vi "FPGA1_EPTDigChannels_ECS.vi"(0 "NI9411-1.2.Filt":u16, 1 "NI9411-1.3.Filt":u16, 2 "NI9411-1.4.Filt":u16, 3 "NI9411-1.5.Filt":u16, 4 "ADCombo-1.VRHallData":T1, 5 "ADCombo-1.VR1.Filt":u16, 6 "ADCombo-1.VR2.Filt":u16, 8 "9411/DI5:0":u8, 9 "ADCombo-1.Hall1.Filt":u16, 10 "NI9411-1.1.Filt":u16, 11 "ADCombo-1.Hall2.Filt":u16, 12 "NI9411-1.Invert":u8, 13 "ADCombo-1.VRHallInvert":u8, 14 "NI9411-1.0.Filt":u16) -> (16 "9411-1.0.PPWData":T2, 17 "ADCombo-1.Hall2.PPWData":T2, 18 "9411-1.1.PPWData":T2, 19 "ADCombo-1.Hall1.PPWData":T2, 20 "9411-1.2.PPWData":T2, 21 "9411-1.3.PPWData":T2, 22 "9411-1.4.PPWData":T2, 23 "9411-1.5.PPWData":T2, 24 "9411-1.DigitalTriggers":bool[](array[boolean]), 25 "ADCombo-1.VR1.PPWData":T2, 26 "ADCombo-1.VR2.PPWData":T2, 27 "ADCombo-1.DigitalTriggers":bool[](array[boolean]))   [LabVIEW 2015, in "ECS-FPGA.lvlib"]
uses:
  ECS-FPGA.lvlib
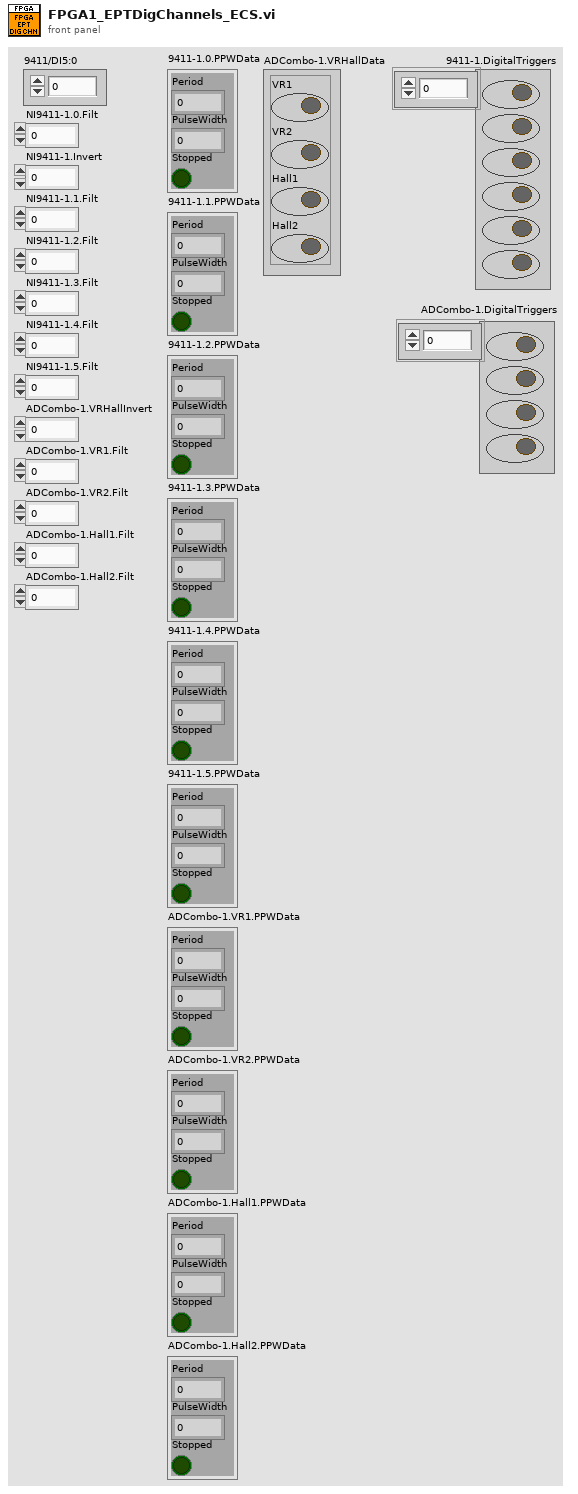
[diagram p1: front panel]
types:
  T1 = cluster{"VR1":bool, "VR2":bool, "Hall1":bool, "Hall2":bool}
  T2 = cluster{"Period":u32, "PulseWidth":u32, "Stopped":bool}
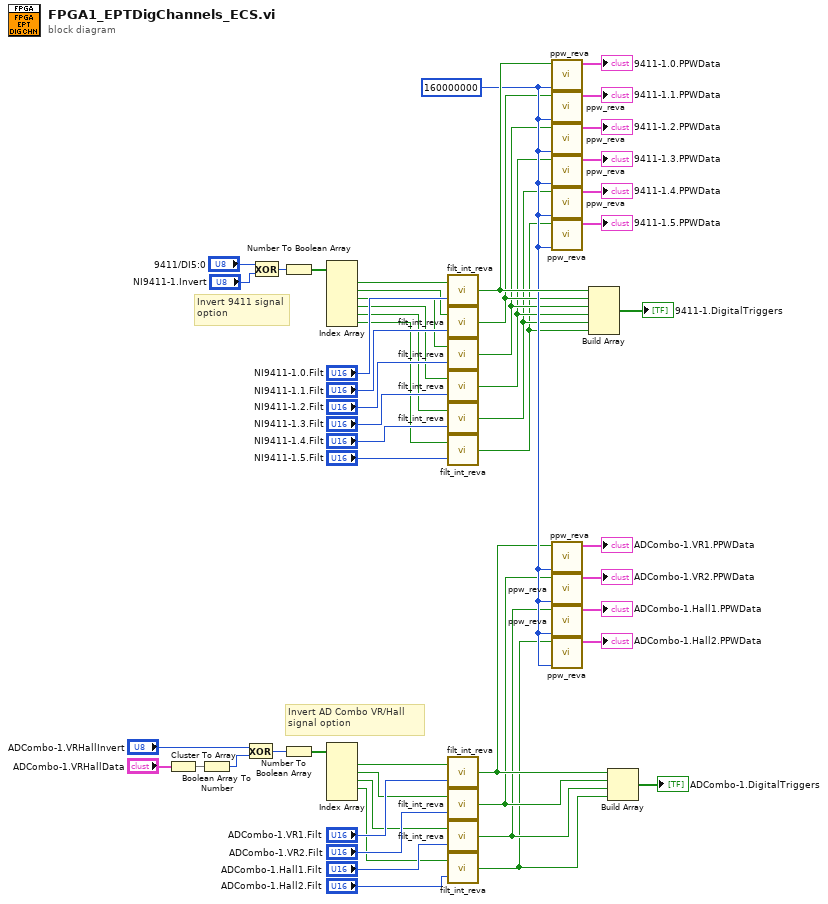
[diagram p0: block diagram]
diagram:
  w48 = u32 160000000 ("StopValue")
  # "Invert AD Combo VR/Hall\nsignal option"
  # "Invert 9411 signal\noption"
  n1 = Cluster To Array(cluster="ADCombo-1.VRHallData") -> (array=w14:bool[])
  n2 = Boolean Array To Number(Boolean array=w14) -> (number=w13:u8)
  n3 = Exclusive Or(1:w13, 2:"ADCombo-1.VRHallInvert") -> (0:w11:u8)
  n4 = Exclusive Or(1:"NI9411-1.Invert", 2:"9411/DI5:0") -> (0:w21:u8)
  n5 = Number To Boolean Array(number=w21) -> (Boolean array=w23:bool[])
  n6 = Number To Boolean Array(number=w11) -> (Boolean array=w9:bool[])
  n7 = Index Array(array=w23) -> (element #1=w24:bool, element #2=w25:bool, element #3=w26:bool, element #4=w27:bool, element #5=w28:bool, element #6=w29:bool)  [unwired: 6 in]
  n8 = Index Array(array=w9) -> (element #1=w10:bool, element #2=w8:bool, element #3=w7:bool, element #4=w6:bool)  [unwired: 5 in, 1 out]
  n9 = call <vilib>:"filt_int_reva.vi"("FiltValue"="NI9411-1.0.Filt", "InpSig"=w24) -> ("OutSig"=w53:bool)
  n10 = call <vilib>:"filt_int_reva.vi"("FiltValue"="NI9411-1.1.Filt", "InpSig"=w25) -> ("OutSig"=w20:bool)
  n11 = call <vilib>:"filt_int_reva.vi"("FiltValue"="NI9411-1.2.Filt", "InpSig"=w26) -> ("OutSig"=w19:bool)
  n12 = call <vilib>:"filt_int_reva.vi"("FiltValue"="NI9411-1.3.Filt", "InpSig"=w27) -> ("OutSig"=w18:bool)
  n13 = call <vilib>:"filt_int_reva.vi"("FiltValue"="NI9411-1.4.Filt", "InpSig"=w28) -> ("OutSig"=w17:bool)
  n14 = call <vilib>:"filt_int_reva.vi"("FiltValue"="NI9411-1.5.Filt", "InpSig"=w29) -> ("OutSig"=w16:bool)
  n15 = call <vilib>:"filt_int_reva.vi"("FiltValue"="ADCombo-1.VR1.Filt", "InpSig"=w10) -> ("OutSig"=w5:bool)
  n16 = call <vilib>:"filt_int_reva.vi"("FiltValue"="ADCombo-1.VR2.Filt", "InpSig"=w8) -> ("OutSig"=w4:bool)
  n17 = call <vilib>:"filt_int_reva.vi"("FiltValue"="ADCombo-1.Hall1.Filt", "InpSig"=w7) -> ("OutSig"=w3:bool)
  n18 = call <vilib>:"filt_int_reva.vi"("FiltValue"="ADCombo-1.Hall2.Filt", "InpSig"=w6) -> ("OutSig"=w2:bool)
  n19 = call <vilib>:"ppw_reva.vi"("StopValue"=w48, "InpSig"=w53) -> ("PPWData"=→"9411-1.0.PPWData":T2)  [unwired: 2 in, 3 out]
  n20 = call <vilib>:"ppw_reva.vi"("StopValue"=w48, "InpSig"=w20) -> ("PPWData"=→"9411-1.1.PPWData":T2)  [unwired: 2 in, 3 out]
  n21 = call <vilib>:"ppw_reva.vi"("StopValue"=w48, "InpSig"=w19) -> ("PPWData"=→"9411-1.2.PPWData":T2)  [unwired: 2 in, 3 out]
  n22 = call <vilib>:"ppw_reva.vi"("StopValue"=w48, "InpSig"=w18) -> ("PPWData"=→"9411-1.3.PPWData":T2)  [unwired: 2 in, 3 out]
  n23 = call <vilib>:"ppw_reva.vi"("StopValue"=w48, "InpSig"=w17) -> ("PPWData"=→"9411-1.4.PPWData":T2)  [unwired: 2 in, 3 out]
  n24 = call <vilib>:"ppw_reva.vi"("StopValue"=w48, "InpSig"=w16) -> ("PPWData"=→"9411-1.5.PPWData":T2)  [unwired: 2 in, 3 out]
  n25 = call <vilib>:"ppw_reva.vi"("StopValue"=w48, "InpSig"=w5) -> ("PPWData"=→"ADCombo-1.VR1.PPWData":T2)  [unwired: 2 in, 3 out]
  n26 = call <vilib>:"ppw_reva.vi"("StopValue"=w48, "InpSig"=w4) -> ("PPWData"=→"ADCombo-1.VR2.PPWData":T2)  [unwired: 2 in, 3 out]
  n27 = call <vilib>:"ppw_reva.vi"("StopValue"=w48, "InpSig"=w3) -> ("PPWData"=→"ADCombo-1.Hall1.PPWData":T2)  [unwired: 2 in, 3 out]
  n28 = call <vilib>:"ppw_reva.vi"("StopValue"=w48, "InpSig"=w2) -> ("PPWData"=→"ADCombo-1.Hall2.PPWData":T2)  [unwired: 2 in, 3 out]
  n29 = Build Array(w53, w20, w19, w18, w17, w16) -> (→"9411-1.DigitalTriggers":bool[])
  n30 = Build Array(w5, w4, w3, w2) -> (→"ADCombo-1.DigitalTriggers":bool[])
